vi "IX83 Controller.vi"() -> ()   [LabVIEW 2017]
panel:
  in  "SendCommand":bool
  out "Response":string
  in  "Stop":bool
  out "CONNECTING":bool
  in  "Command":string
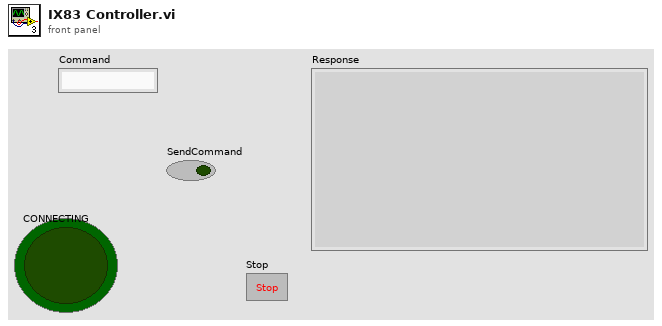
[diagram p1: front panel]
types:
  T1 = enum16{"Standard", "Buffered", "CRLF", "Immediate"}
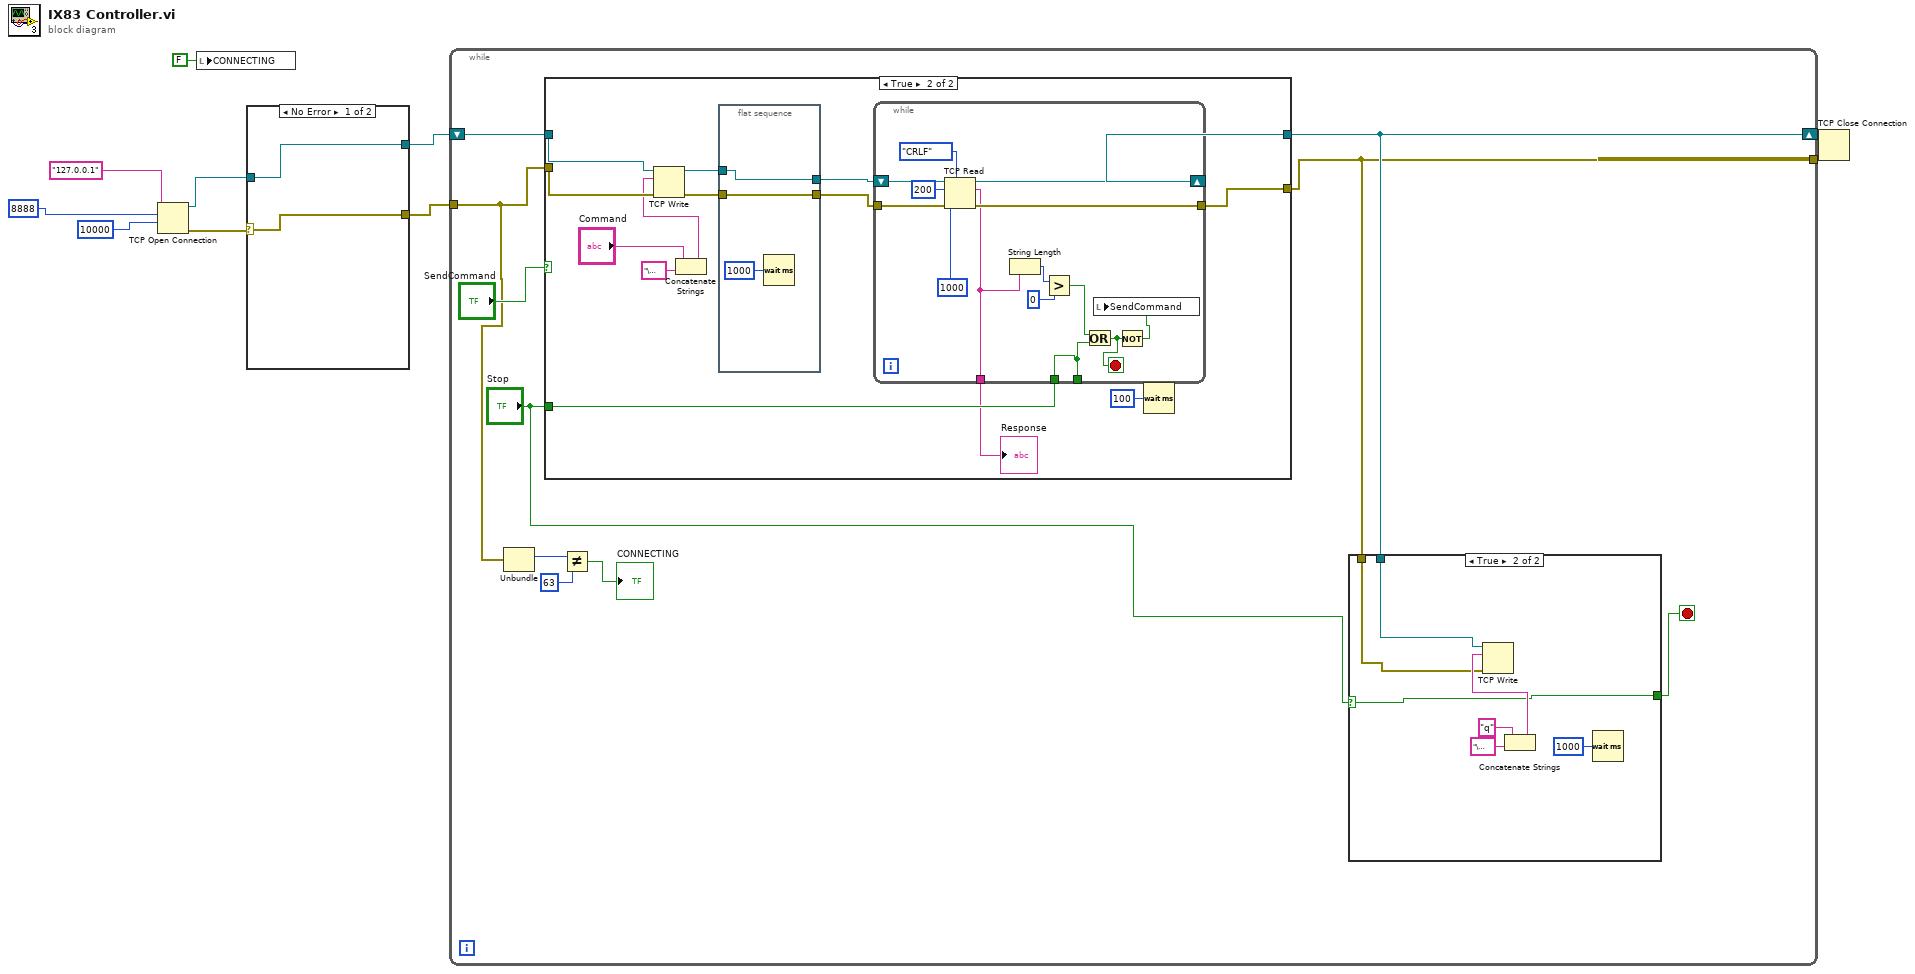
[diagram p0: block diagram]
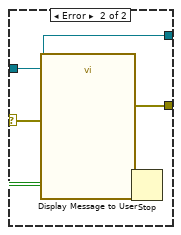
[diagram p2: hidden frame]
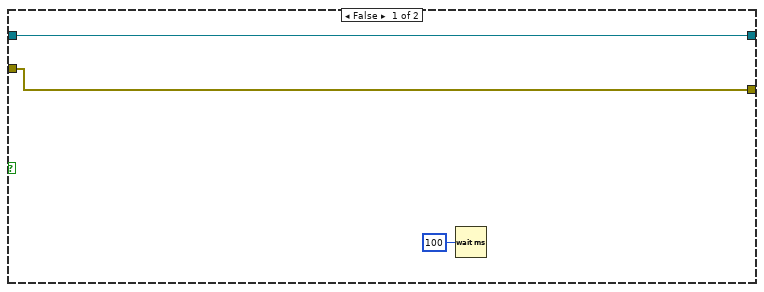
[diagram p4: hidden frame]
diagram:
  n1 = TCP Open Connection(address="127.0.0.1" ("服务名称"), remote port or service name=u16 8888 ("端口"), timeout ms (60000)=10000) -> (connection ID=w3:refnum<k5>, error out=w4:errorcluster)  [unwired: 2 in]
  n2 = local write "CONNECTING"(FALSE ("CONNECTING")) -> ()
  n3 = case shown="No Error" w4 {
    selector: w4 -> [w11 w15]
    tunnel: w3 -> [w12 w14]
    tunnel: [w12 w14] -> w2
    tunnel: [w11 w15] -> w1
    frame No Error {
    }
    frame Error {
      n4 = call "Display Message to User"() -> ("OK"=w13:bool)  [unwired: 10 in, 1 out]
      n5 = Stop(stop? (T)=w13) -> ()
    }
  }
  n6 = while {
    shift-right: [w17] -> w10
    shift-left: w2 -> [w25]
    tunnel: [w16] -> w7
    tunnel: w1 -> [w21]
    stop <- w18 stop-if-true
    n7 = Unbundle(w21) -> ("code"=w23:i32)  [unwired: 2 out]
    n8 = case shown="True" "SendCommand" {
      tunnel: w25 -> [w36 w50]
      tunnel: [w36 w49] -> w17
      tunnel: [w35 w48] -> w16
      tunnel: w21 -> [w35 w47]
      tunnel: "Stop" -> [_ w46]
      frame False {
        n9 = Wait (ms)(milliseconds to wait=u32 100 ("等待时间（毫秒）")) -> ()  [unwired: 1 out]
      }
      frame True {
        n10 = Concatenate Strings("Command", "\u0000" ("string")) -> (w44:string)
        n11 = TCP Write(connection ID=w50, data in=w44, error in (no error)=w47) -> (connection ID out=w40:refnum<k5>, error out=w38:errorcluster)  [unwired: 1 in, 1 out]
        n12 = flat-sequence {
          tunnel: [w53] -> w41
          tunnel: w40 -> [w53]
          tunnel: [w52] -> w39
          tunnel: w38 -> [w52]
          frame #0 {
            n13 = Wait (ms)(milliseconds to wait=u32 1000 ("等待时间（毫秒）")) -> ()  [unwired: 1 out]
          }
        }
        n14 = while {
          shift-right: [w66] -> w49
          shift-left: w41 -> [w67]
          tunnel: [w62] -> w48
          tunnel: [w60] -> _
          tunnel: w39 -> [w61]
          tunnel: w46 -> [w60]
          tunnel: [w56] -> w43
          stop <- w55 stop-if-true
          n15 = TCP Read(connection ID=w67, bytes to read=200 ("读取的字节"), error in (no error)=w61, 7:T1."CRLF" ("模式（标准）"), 9:1000 ("超时毫秒(25000)")) -> (connection ID out=w66:refnum<k5>, data out=w56:string, error out=w62:errorcluster)
          n16 = String Length(string=w56) -> (length=w65:i32)
          n17 = Greater?(x=w65, y=0) -> (0:w63:bool)
          n18 = Or(x=w63, y=w60) -> (x .or. y?=w55:bool)
          n19 = Not(x=w55) -> (.not. x?=w54:bool)
          n20 = local write "SendCommand"(w54) -> ()
        }
        "Response" <- w43
        n21 = Wait (ms)(milliseconds to wait=u32 100 ("等待时间（毫秒）")) -> ()  [unwired: 1 out]
      }
    }
    n22 = Not Equal?(x=w23, y=63) -> (x != y?=→"CONNECTING":bool)
    n23 = case shown="True" "Stop" {
      selector: "Stop" -> [w26 w30]
      tunnel: [w26 w30] -> w18
      tunnel: w17 -> [_ w29]
      tunnel: w16 -> [_ w28]
      frame False {
      }
      frame True {
        n24 = Concatenate Strings("q" ("string"), "\u0000" ("string")) -> (w33:string)
        n25 = TCP Write(connection ID=w29, data in=w33, error in (no error)=w28) -> ()  [unwired: 1 in, 3 out]
        n26 = Wait (ms)(milliseconds to wait=u32 1000 ("等待时间（毫秒）")) -> ()  [unwired: 1 out]
      }
    }
  }
  n27 = TCP Close Connection(connection ID=w10, error in (no error)=w7) -> ()  [unwired: 1 in, 2 out]
